vi "DefesaAntigaAdaptada.vi"(0 "Our Robot":T1={"id"=0, "function"=enum."Attacker", "x"=0.0, "y"=0.0, "orientation"=0.0, "v_tangent"=0.0, "v_normal"=0.0, "v_ang"=0.0, "kick_x"=0.0, "kick_z"=0.0, "dribble"=FALSE, "Timestamp"=timestamp(0 s since 1904-01-01), "estimatives"={"est_v_tangent"=0.0, "est_v_normal"=0.0, "est_vx"=0.0, "est_vy"=0.0, "Pos Robot Est"=[]}, "dest_x_kick"=0.0, "dest_y_kick"=0.0, "Gap Coord"=[], "States"=enum."GoToTangent", "Path "=[], "Path  Smooth"=[], "Dest"=[]}, 1 "total de \ndefensores":i32, 3 "Stop?":bool=TRUE, 4 "AI Parameters":T12={"GotoKick"={"Dist do cone a frente"=150.0, "attacker farback"=1500.0, "Perto"=300.0, "min dist to kick"=150.0, "kick eps"=0.0, "Time to transition"=0.05}, "Attacker"={"CC chute"=0.09, "CC passe"=0.045, "Kick Force"=100.0, "D ball-robot Kick"=200.0, "D ball-robot Pass"=0.3}, "Defender"={"D max"=1700.0, "Vel p/ robô av"=1000.0, "Kick Force"=100.0, "D atk-def"=0.0, "D farback"=0.0}, "Timeout"={"Field/v in x"=6.0, "Dist Robots"=300, "Dist up in y"=300}, "Pose Striker"={"dist"=200.0, "Numeric"=-4.0, "dist 2"=200.0}, "Dist Stop"=300.0, "Distance when ball out"=200, "D central gap "=150.0, "T pass"=0.0, "Force ++"=0.0, "range kick"=0.0, "Chute alto"=TRUE, "Marcador novo"=TRUE} {"D central gap" format="%#_13g"; "Dist Stop" format="%#_13g"; "Pose Striker"."Numeric" format="%#_13g"; "Defender"."Kick Force" format="%#_13g"; "Defender"."Vel p/ robô av" format="%#_13g"; "Attacker"."D ball-robot Kick" format="%#_13g"; "Attacker"."Kick Force" format="%#_13g"; "Attacker"."CC passe" format="%#_13g"; "Attacker"."CC chute" format="%#_13g"; "GotoKick"."kick eps" format="%#_13g"; "GotoKick"."min dist to kick" format="%#_13g"; "GotoKick"."Perto" format="%#_13g"; "GotoKick"."attacker farback" format="%#_13g"; "GotoKick"."Dist do cone a frente" format="%#_13g"}, 5 "balls":T7[](array[typedef]), 9 "geometry":T8, 10 "Atacando contra?":bool=TRUE, 11 "Field defense":dbl[](array[numeric]), 12 "Defensores":u32[](array[numeric]), 14 "IA State Input 2":T6={"our_robots"=[], "enemy_robots"=[], "balls"=[], "geometry"={"line_width"=0, "field_length"=0, "field_width"=0, "boundary_width"=0, "referee_width"=0, "goal_width"=0, "goal_depth"=0, "goal_wall_width"=0, "center_circle_radius"=0, "defense_radius"=0, "defense_stretch"=0, "free_kick_from_defense_dist"=0, "penalty_spot_from_field_line_dist"=0, "penalty_line_from_spot_dist"=0}, "IA Judge"={"stage"="", "command"="", "our_goalie_id"=0.0, "enemy_goalie_id"=0.0, "command enum"=enum."Halt", "Time"=enum."Azul"}, "Received Timestamp"=timestamp(0 s since 1904-01-01), "Events"={"Touch"=FALSE, "Ball out"=FALSE, "id touch"=0.0, "Ball out of \nVision"=FALSE, "Ball inside \nGoalie area"=FALSE, "Robot not responding"=FALSE, "Robots responding status"=[1.0, 1.0, 1.0, 1.0, 1.0, 1.0], "Enemy Ball \nPossession"=FALSE, "Pass State"=FALSE, "id end of pass"=0.0, "Kick"=FALSE, "Id ini Possession"=0.0, "Ball Possesion"=FALSE, "Id Possesion"=0.0}}) -> (2 "Id duelist":i32, 6 "Robot out":T1={"id"=0, "function"=enum."Attacker", "x"=0.0, "y"=0.0, "orientation"=0.0, "v_tangent"=0.0, "v_normal"=0.0, "v_ang"=0.0, "kick_x"=0.0, "kick_z"=0.0, "dribble"=FALSE, "Timestamp"=timestamp(0 s since 1904-01-01), "estimatives"={"est_v_tangent"=0.0, "est_v_normal"=0.0, "est_vx"=0.0, "est_vy"=0.0, "Pos Robot Est"=[]}, "dest_x_kick"=0.0, "dest_y_kick"=0.0, "Gap Coord"=[], "States"=enum."GoToTangent", "Path "=[], "Path  Smooth"=[], "Dest"=[]}, 13 "Zageuiro duelist?":bool=TRUE)   [LabVIEW 2017]
uses:
  AI Parameters.ctl
  Core/AI Robot.ctl
  Functions Enum.ctl
  AttackerStates.ctl
  Path Planning/RRT/PathDests.ctl
  Path Planning/RRT/PathDest.ctl
  Core/Field Size.ctl
  Core/AI Ball.ctl
  Core/AI Input.ctl
  Core/AI Judge.ctl
  Command Enum.ctl
  Util/Events/Events.ctl
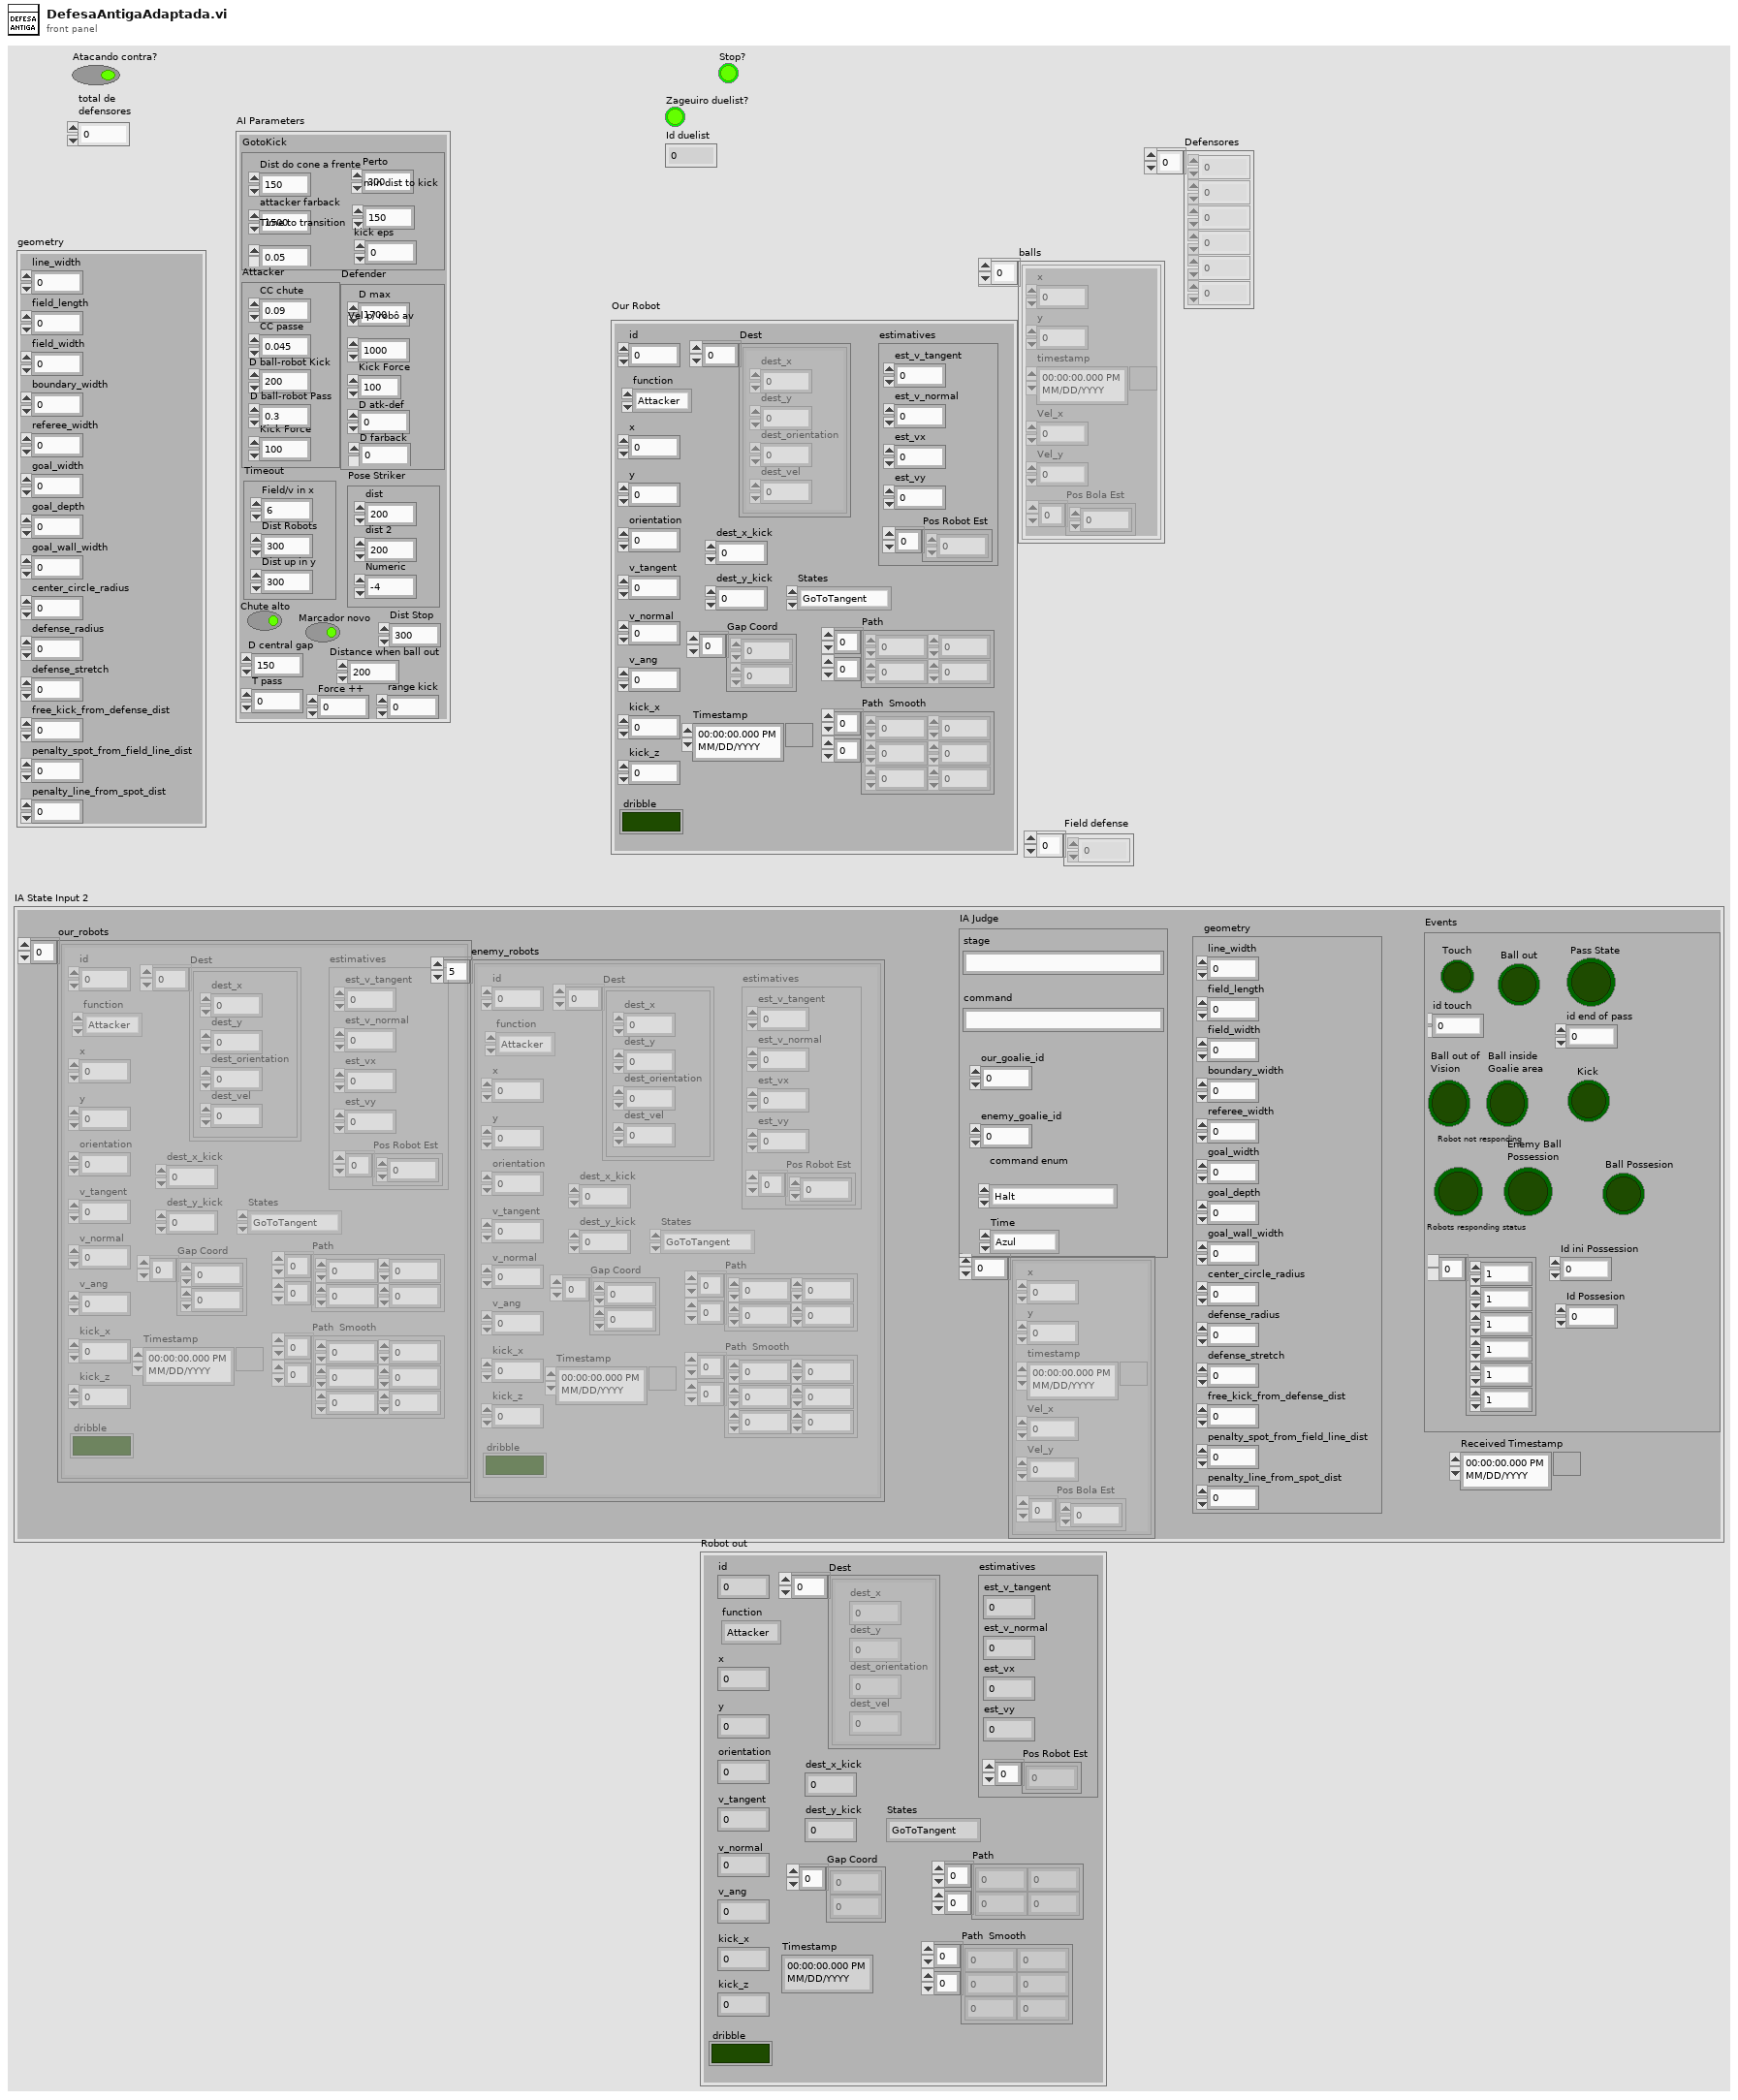
[diagram p1: front panel]
types:
  T1 = typedef "AI Robot.ctl" = cluster{"id":u32, "function":T2, "x":dbl, "y":dbl, "orientation":dbl, "v_tangent":dbl, "v_normal":dbl, "v_ang":dbl, "kick_x":dbl, "kick_z":dbl, "dribble":bool, "Timestamp":timestamp, "estimatives":cluster{"est_v_tangent":dbl, "est_v_normal":dbl, "est_vx":dbl, "est_vy":dbl, "Pos Robot Est":dbl[]}, "dest_x_kick":dbl, "dest_y_kick":dbl, "Gap Coord":dbl[], "States":T3, "Path ":dbl[][], "Path  Smooth":dbl[][], "Dest":T4}
  T2 = typedef "Functions Enum.ctl" = enum16{"Attacker", "Goalie", "Defender", "Striker", "Goto 0", "Dummy", "Kicker", "ZigZag"}
  T3 = typedef "AttackerStates.ctl" = enum16{"Pass", "GoToTangent", "BallGetting", "GoToKick", ""}
  T4 = typedef "PathDests.ctl" = T5[]
  T5 = typedef "PathDest.ctl" = cluster{"dest_x":dbl, "dest_y":dbl, "dest_orientation":dbl, "dest_vel":dbl}
  T6 = typedef "AI Input.ctl" = cluster{"our_robots":T1[], "enemy_robots":T1[], "balls":T7[], "geometry":T8, "IA Judge":T9, "Received Timestamp":timestamp, "Events":T11}
  T7 = typedef "AI Ball.ctl" = cluster{"x":dbl, "y":dbl, "timestamp":timestamp, "Vel_x":dbl, "Vel_y":dbl, "Pos Bola Est":dbl[]}
  T8 = typedef "Field Size.ctl" = cluster{"line_width":u32, "field_length":u32, "field_width":u32, "boundary_width":u32, "referee_width":u32, "goal_width":u32, "goal_depth":u32, "goal_wall_width":u32, "center_circle_radius":u32, "defense_radius":u32, "defense_stretch":u32, "free_kick_from_defense_dist":u32, "penalty_spot_from_field_line_dist":u32, "penalty_line_from_spot_dist":u32}
  T9 = typedef "AI Judge.ctl" = cluster{"stage":string, "command":string, "our_goalie_id":dbl, "enemy_goalie_id":dbl, "command enum":T10, "Time":enum16{"Azul", "Amarelo"}}
  T10 = typedef "Command Enum.ctl" = enum16{"Halt", "Stop", "Force Start", "PKA Normal Start", "Prepare Kickoff Ally", "PKE Normal Start", "Prepare Kickoff Enemy", "Prepare Penalty Ally", "PPA Normal Start", "Prepare Penalty Enemy", "PPE Normal Start", "Direct Free Enemy", "Direct Free Ally", "Indirect Free Enemy", "Indirect Free Ally", "Timeout Enemy", "Timeout Ally", "Goal Enemy", "Goal Ally", "Ball Placement Enemy", "Ball Placement Ally", "Normal Half Time", "Extra Time Break", "Extra Half Time", "None", "Post Game"}
  T11 = typedef "Events.ctl" = cluster{"Touch":bool, "Ball out":bool, "id touch":dbl, "Ball out of \nVision":bool, "Ball inside \nGoalie area":bool, "Robot not responding":bool, "Robots responding status":dbl[], "Enemy Ball \nPossession":bool, "Pass State":bool, "id end of pass":dbl, "Kick":bool, "Id ini Possession":dbl, "Ball Possesion":bool, "Id Possesion":dbl}
  T12 = typedef "AI Parameters.ctl" = cluster{"GotoKick":cluster{"Dist do cone a frente":dbl, "attacker farback":dbl, "Perto":dbl, "min dist to kick":dbl, "kick eps":dbl, "Time to transition":dbl}, "Attacker":cluster{"CC chute":dbl, "CC passe":dbl, "Kick Force":dbl, "D ball-robot Kick":dbl, "D ball-robot Pass":dbl}, "Defender":cluster{"D max":dbl, "Vel p/ robô av":dbl, "Kick Force":dbl, "D atk-def":dbl, "D farback":dbl}, "Timeout":cluster{"Field/v in x":dbl, "Dist Robots":u32, "Dist up in y":u32}, "Pose Striker":cluster{"dist":dbl, "Numeric":dbl, "dist 2":dbl}, "Dist Stop":dbl, "Distance when ball out":i32, "D central gap ":dbl, "T pass":dbl, "Force ++":dbl, "range kick":dbl, "Chute alto":bool, "Marcador novo":bool}
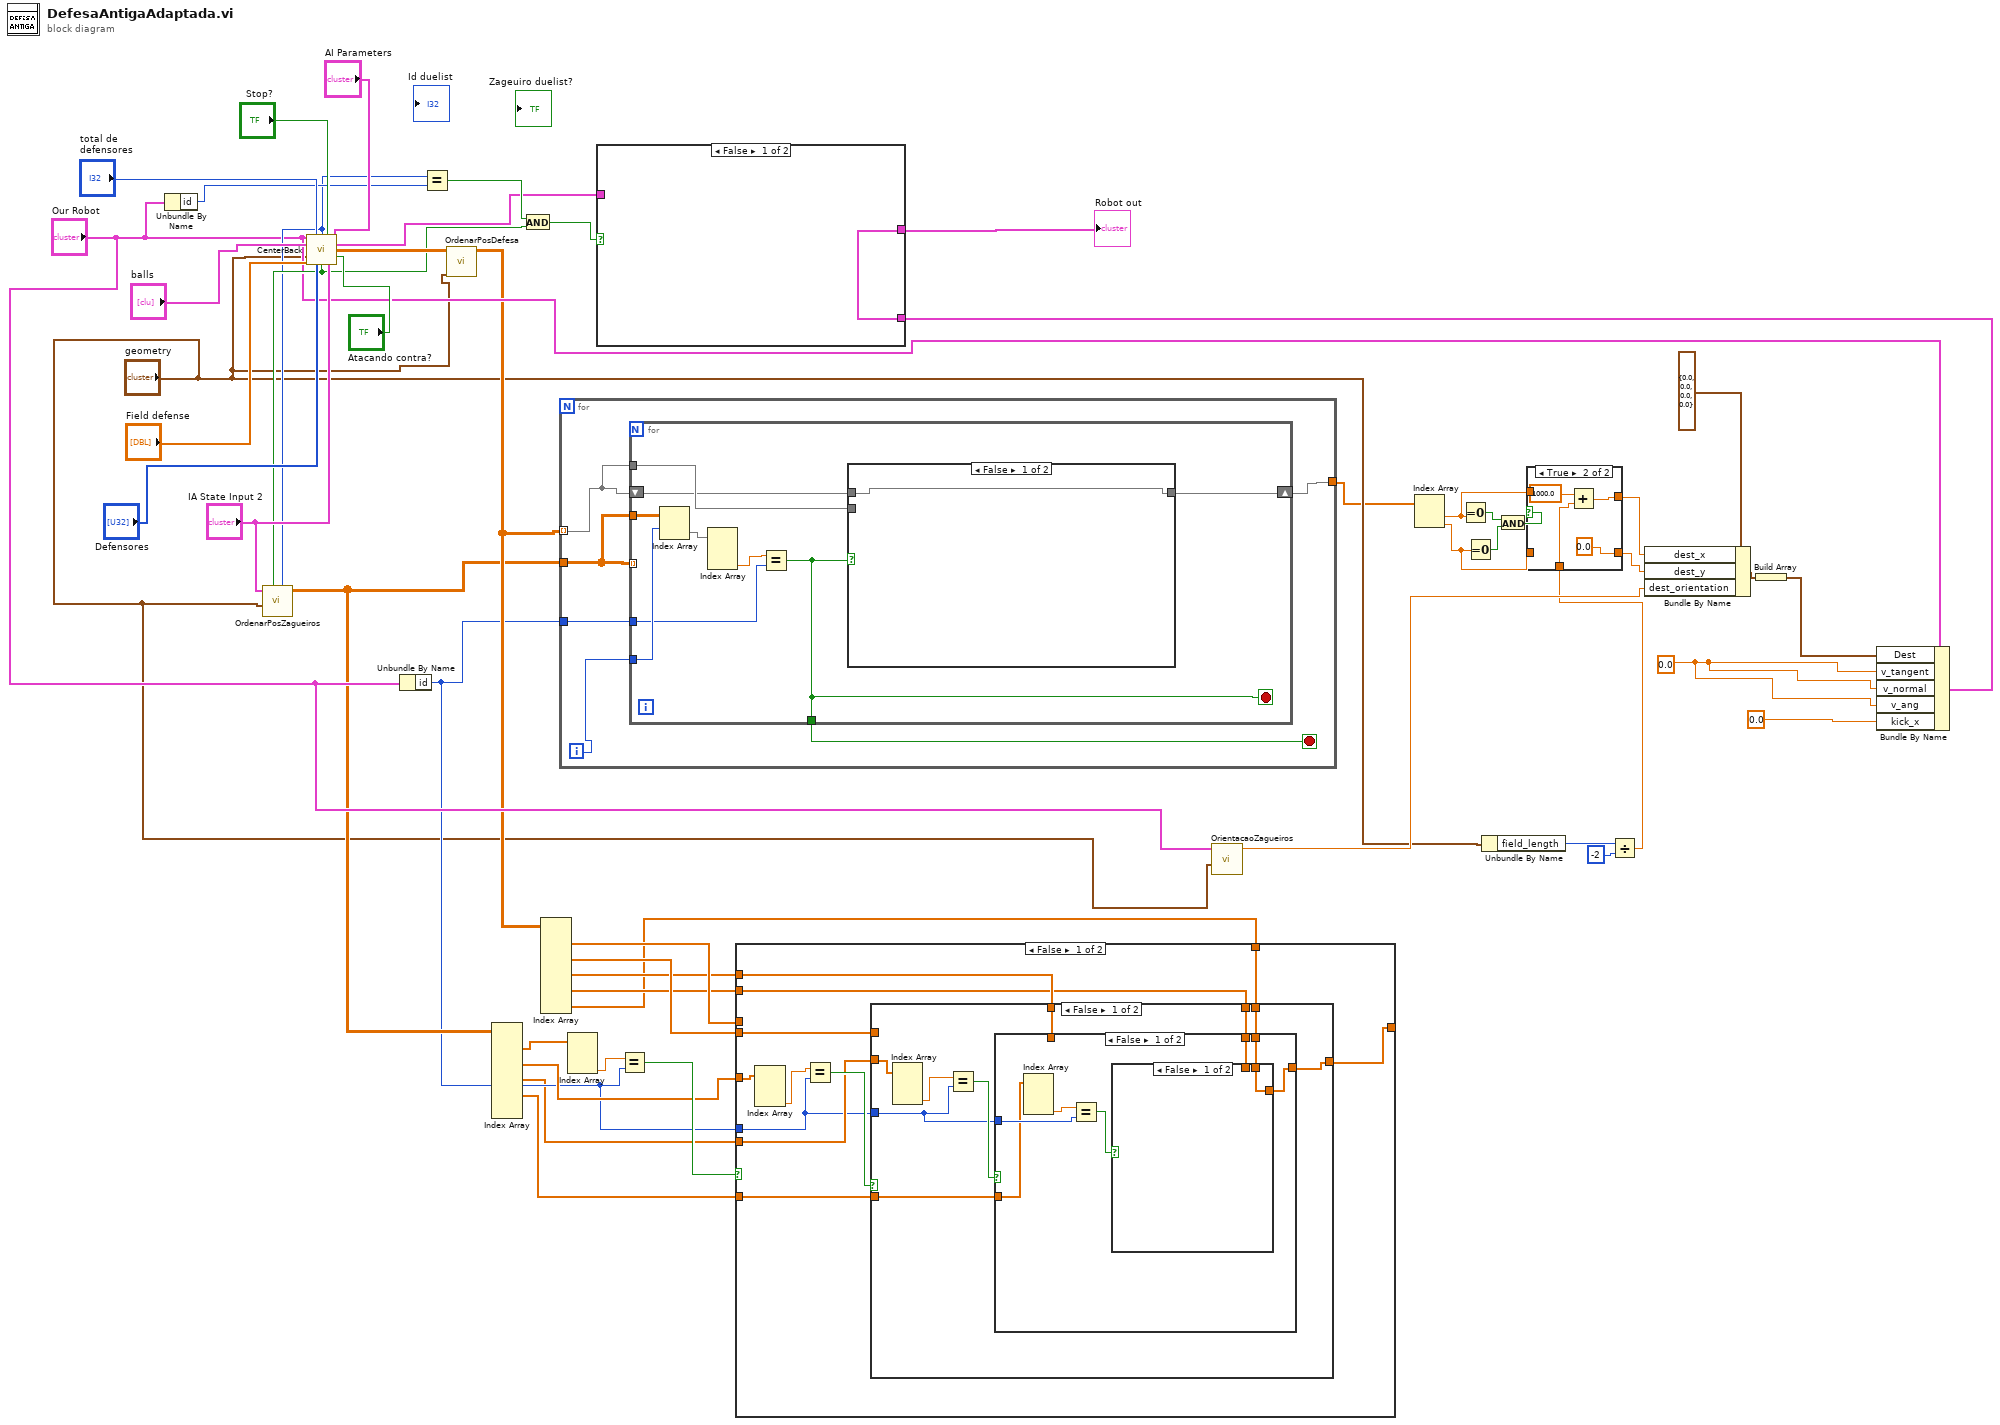
[diagram p0: block diagram]
diagram:
  w27 = 0.0
  n1 = Unbundle By Name("Our Robot") -> ("id"=w42:u32)
  n2 = call "CenterBack.vi"("Our Robot in"="Our Robot", "total"="total de \ndefensores", "Stop?"="Stop?", "AI Parameters"="AI Parameters", "balls"="balls", "Field Size in"="geometry", "Atacando contra?"="Atacando contra?", "Field defense"="Field defense", "Defensores"="Defensores", "IA State Input 2"="IA State Input 2") -> ("Id duelist"=w35:i32, "Robot out"=w38:T1, "Pos Centers Back"=w50:dbl[][], "Zageuiro duelist?"=w36:bool)  [unwired: 2 in]
  n3 = call "OrdenarPosZagueiros.vi"("ID duelist"=w35, "Zagueiro duelist?"=w36, "geometry"="geometry", "IA State Input 2"="IA State Input 2") -> ("Posições ordenadas zagueiros"=w25:dbl[][])  [unwired: 7 in]
  n4 = Unbundle By Name("Our Robot") -> ("id"=w19:u32)
  n5 = Equal?(x=w35, y=w42) -> (x = y?=w41:bool)
  n6 = call "OrdenarPosDefesa.vi"("geometry"="geometry", "Posições da defesa"=w50) -> ("Posições ordenadas"=w26:dbl[][])  [unwired: 9 in]
  n7 = Index Array(array=w25) -> (element #1=w24:dbl[], element #2=w20:dbl[], element #3=w17:dbl[], element #4=w15:dbl[])  [unwired: 10 in, 1 out]
  n8 = And(x=w41, y=w36) -> (x .and. y?=w40:bool)
  n9 = Index Array(array=w26) -> (element #1=w21:dbl[], element #2=w18:dbl[], element #3=w16:dbl[], element #4=w14:dbl[], element #5=w13:dbl[])  [unwired: 10 in]
  n10 = for {
    tunnel: w26 -> [w53] mode=indexing
    tunnel: w25 -> [w55]
    tunnel: w19 -> [w56]
    tunnel: [w52] -> w1
    i -> [w54]
    stop <- w51 stop-if-true
    n11 = for {
      tunnel: w55 -> [_] mode=indexing
      tunnel: w56 -> [w61]
      tunnel: w55 -> [w65]
      tunnel: w54 -> [w64]
      shift-right: [w59] -> w52
      shift-left: w53 -> [w58]
      tunnel: w53 -> [w60]
      tunnel: [w57] -> w51
      stop <- w57 stop-if-true
      n12 = Index Array(array=w65, index (row)=w64) -> (element=w63:dbl[])  [unwired: 1 in]
      n13 = Index Array(array=w63) -> (element #3=w62:dbl)  [unwired: 3 in, 2 out]
      n14 = Equal?(x=w62, y=w61) -> (x = y?=w57:bool)
      n15 = case shown="False" w57 {
        tunnel: w60 -> [_ w67]
        tunnel: [w66 w67] -> w59
        tunnel: w58 -> [w66 _]
        frame False {
        }
        frame True {
        }
      }
    }
  }
  n16 = Index Array(array=w24) -> (element #3=w23:dbl)  [unwired: 3 in, 2 out]
  n17 = Equal?(x=w23, y=w19) -> (x = y?=w22:bool)
  n18 = case shown="False" w22 {
    tunnel: [w75 w99] -> _
    tunnel: w21 -> [_ w99]
    tunnel: w20 -> [w78 _]
    tunnel: w19 -> [w72 _]
    tunnel: w18 -> [w74 _]
    tunnel: w17 -> [w73 _]
    tunnel: w16 -> [w71 _]
    tunnel: w15 -> [w70 _]
    tunnel: w14 -> [w69 _]
    tunnel: w13 -> [w68 _]
    frame False {
      n19 = Index Array(array=w78) -> (element #3=w77:dbl)  [unwired: 3 in, 2 out]
      n20 = Equal?(x=w77, y=w72) -> (x = y?=w76:bool)
      n21 = case shown="False" w76 {
        tunnel: [w84 w98] -> w75
        tunnel: w74 -> [_ w98]
        tunnel: w73 -> [w87 _]
        tunnel: w72 -> [w82 _]
        tunnel: w71 -> [w83 _]
        tunnel: w70 -> [w81 _]
        tunnel: w69 -> [w80 _]
        tunnel: w68 -> [w79 _]
        frame False {
          n22 = Index Array(array=w87) -> (element #3=w86:dbl)  [unwired: 3 in, 2 out]
          n23 = Equal?(x=w86, y=w82) -> (x = y?=w85:bool)
          n24 = case shown="False" w85 {
            tunnel: [w90 w97] -> w84
            tunnel: w83 -> [_ w97]
            tunnel: w82 -> [w94 _]
            tunnel: w81 -> [w92 _]
            tunnel: w80 -> [w89 _]
            tunnel: w79 -> [w88 _]
            frame False {
              n25 = Index Array(array=w92) -> (element #3=w93:dbl)  [unwired: 3 in, 2 out]
              n26 = Equal?(x=w93, y=w94) -> (x = y?=w91:bool)
              n27 = case shown="False" w91 {
                tunnel: [w95 w96] -> w90
                tunnel: w89 -> [_ w96]
                tunnel: w88 -> [w95 _]
                frame False {
                }
                frame True {
                }
              }
            }
            frame True {
            }
          }
        }
        frame True {
        }
      }
    }
    frame True {
    }
  }
  n28 = call "OrientacaoZagueiros.vi"("geometry"="geometry", "Our Robot"="Our Robot") -> ("Orientação Center Back"=w28:dbl)  [unwired: 9 in]
  n29 = Index Array(array=w1) -> (element #1=w8:dbl, element #2=w6:dbl)  [unwired: 2 in]
  n30 = Equal To 0?(x=w8) -> (x = 0?=w12:bool)
  n31 = Equal To 0?(x=w6) -> (x = 0?=w11:bool)
  n32 = Unbundle By Name("geometry") -> ("field_length"=w4:u32)
  n33 = And(x=w12, y=w11) -> (x .and. y?=w10:bool)
  n34 = Divide(x=w4, y=-2) -> (x/y=w2:dbl)
  n35 = case shown="True" w10 {
    tunnel: [w101 w102] -> w9
    tunnel: w8 -> [w101 _]
    tunnel: [w100 0.0] -> w7
    tunnel: w6 -> [w100 _]
    tunnel: w2 -> [_ w104]
    frame False {
    }
    frame True {
      n36 = Add(x=1000.0, y=w104) -> (x+y=w102:dbl)
    }
  }
  n37 = Bundle By Name(cluster=T5 {"dest_x"=0.0, "dest_y"=0.0, "dest_orientation"=0.0, "dest_vel"=0.0} ("element"), "dest_x"=w9, "dest_y"=w7, "dest_orientation"=w28) -> (w34:T5)
  n38 = Build Array(w34) -> (w33:T5[])
  n39 = Bundle By Name(cluster="Our Robot", "Dest"=w33, "v_tangent"=w27, "v_normal"=w27, "v_ang"=w27, "kick_x"=0.0) -> (w30:T1)
  n40 = case shown="False" w40 {
    tunnel: [w106 w107] -> w39
    tunnel: w38 -> [_ w107]
    tunnel: w30 -> [w106 _]
    frame False {
    }
    frame True {
    }
  }
  "Robot out" <- w39
